vi "Hold update .vi"(7 "Enum":enum16{"Read", "Write"}(ring), 8 "error in (no error)":errorcluster, 11 "In":bool) -> (0 "error out":errorcluster, 3 "Out":bool)   [LabVIEW 2022 SP3]
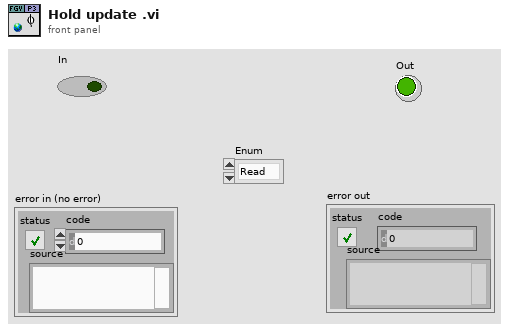
[diagram p1: front panel]
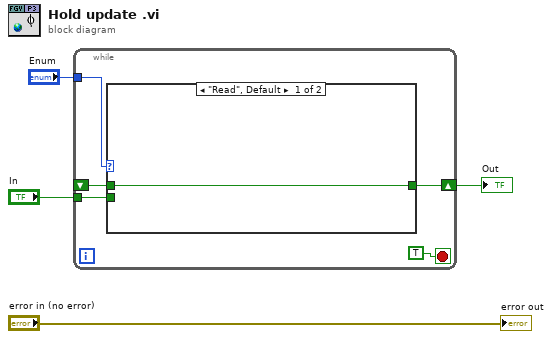
[diagram p0: block diagram]
diagram:
  n1 = while {
    tunnel: "Enum" -> [w8]
    shift-right: [w9] -> w1
    shift-left: _ -> [w7]
    tunnel: "In" -> [w5]
    stop <- TRUE stop-if-true
    n2 = case shown="\"Read\", Default" w8 {
      tunnel: [w10 w11] -> w9
      tunnel: w7 -> [w10 _]
      tunnel: w5 -> [_ w11]
      frame "Read", Default {
      }
      frame "Write" {
      }
    }
  }
  "Out" <- w1
  "error out" <- "error in (no error)"
